vi "upper pop.vi"(1 "pop vi":bool, 2 "error in (no error)":errorcluster, 3 "Feature Selection":T1, 4 "Sub Panel":refnum<vi>) -> (0 "error out":errorcluster)   [LabVIEW 2016, in "main.lvlib"]
doc: "This vi removes whatever vi is running in a sub panel and displays it as a stand alone vi"
uses:
  main.lvlib
  upper subpanel selection.ctl
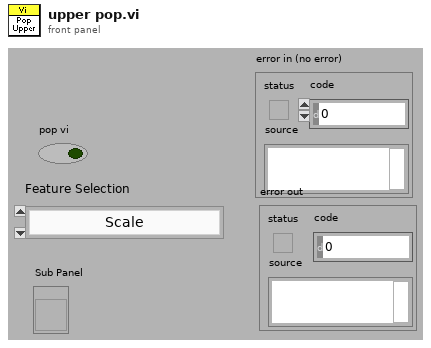
[diagram p1: front panel]
types:
  T1 = typedef "main.lvlib/upper subpanel selection.ctl" = enum16{"Scale", "Injector magnet", "Terminal Voltage", "Source A BPM", "Beam Current", "Flat Top", "Scan Injector", "Scale - old"}
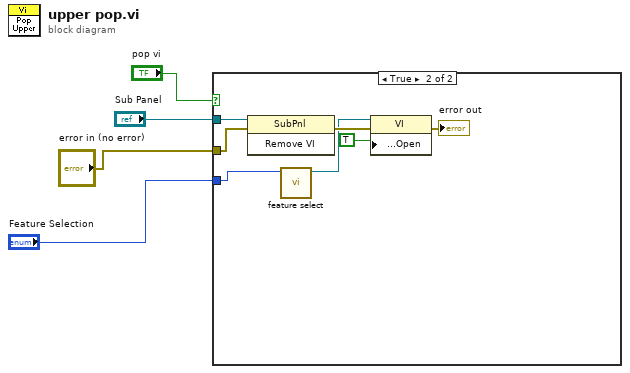
[diagram p0: block diagram]
diagram:
  n1 = case shown="True" "pop vi" {
    tunnel: "Sub Panel" -> [_ w11]
    tunnel: "Feature Selection" -> [_ w6]
    tunnel: "error in (no error)" -> [_ w8]
    frame False {
    }
    frame True {
      n2 = invoke class="SubPnl" method="Remove VI"(reference=w11, error in=w8) -> (error out=w10:errorcluster)  [unwired: 1 in, 2 out]
      n3 = call "feature select.vi"("Feature Selection"=w6) -> ("VI Refnum"=w5:refnum<vi>)  [unwired: 1 in, 7 out]
      n4 = property class="VI"(reference=w5, error in=w10, "Front Panel.Open"=TRUE ("Front Panel Window:Open")) -> (error out=→"error out":errorcluster)  [unwired: 1 out]
    }
  }
